vi "Facade.vi"(0 "Data In":T4, 2 "Display State In":T2, 3 "Container State":T3) -> (6 "Data Out":T4, 7 "Display State Out":T2, 8 "Action":T1)   [LabVIEW 2015, in "Tone (G3).xctl"]
uses:
  Tone (G3).xctl
  Tone.Properties.ctl
  <vilib>/_xctls/Container State.ctl
  State.ctl
  Utility VIs/Controls/KNumeric (DBL)/KNumeric (DBL).xctl
  Utility VIs/Controls/KCheckbox/KCheckbox.xctl
  <vilib>/_xctls/Action.ctl
  <vilib>/_xctls/XControlSupport.lvlib
panel:
  in  "Random phase":bool(xcontrol)
  in  "Frequency (kHz)":dbl(xcontrol)
  in  "Phase (cycles)":dbl(xcontrol)
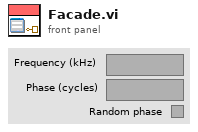
[diagram p1: front panel]
types:
  T1 = typedef "XControlSupport.lvlib/Action.ctl" = cluster{"Data Changed?":bool, "State Changed?":bool, "Action Name":string}
  T2 = typedef "Tone (G3).xctl/State.ctl" = cluster{"enable menu":bool, "ctls":cluster{"Freq":refnum<vi>, "Phase":refnum<vi>, "Random":refnum<vi>}}
  T3 = typedef "XControlSupport.lvlib/Container State.ctl" = cluster{"Indicator?":bool, "Run Mode?":bool, " Refnum":refnum<vi>}
  T4 = typedef "Tone (G3).xctl/Tone.Properties.ctl" = cluster{"Frequency (kHz)":dbl, "Phase (cycles)":dbl, "Random phase":bool}
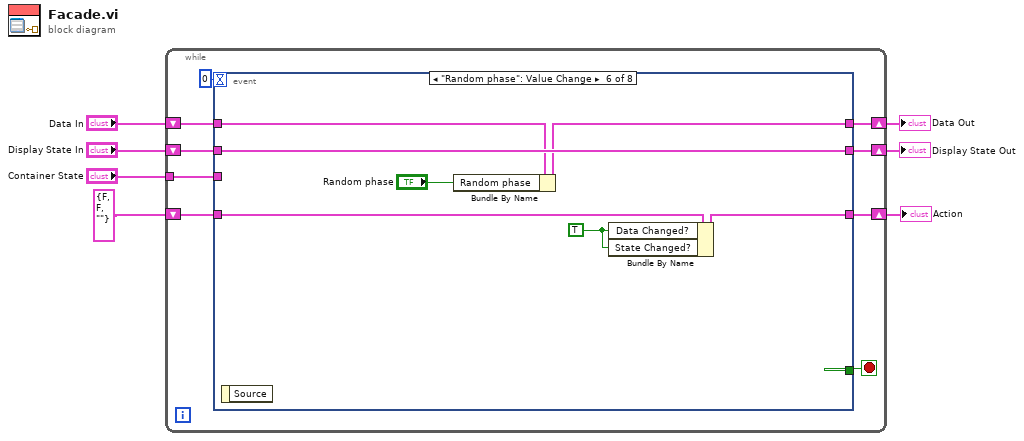
[diagram p0: block diagram]
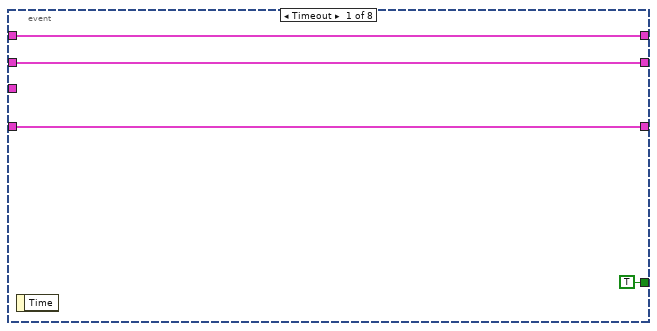
[diagram p2: hidden frame]
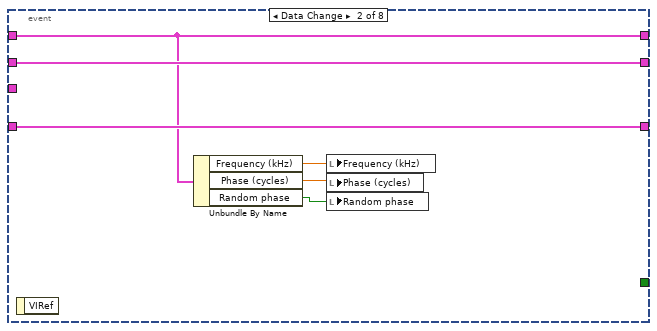
[diagram p3: hidden frame]
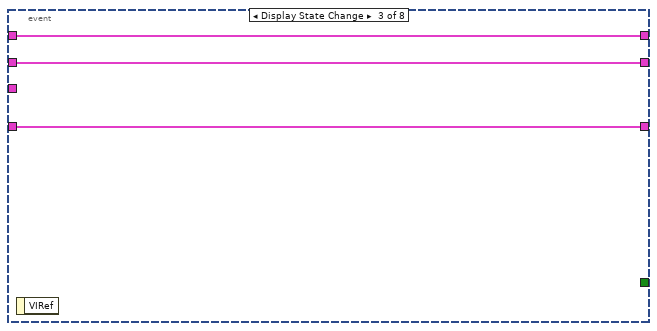
[diagram p4: hidden frame]
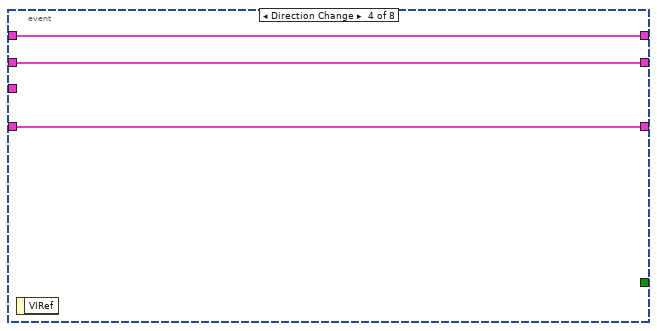
[diagram p5: hidden frame]
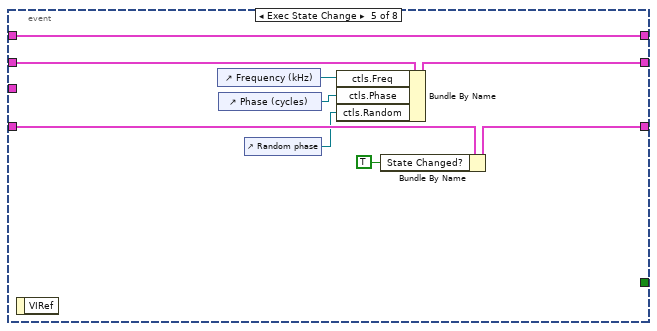
[diagram p6: hidden frame]
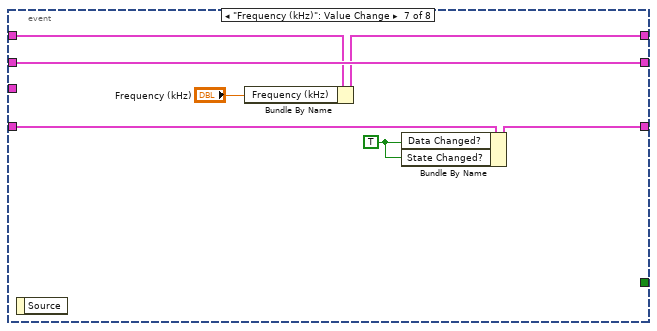
[diagram p7: hidden frame]
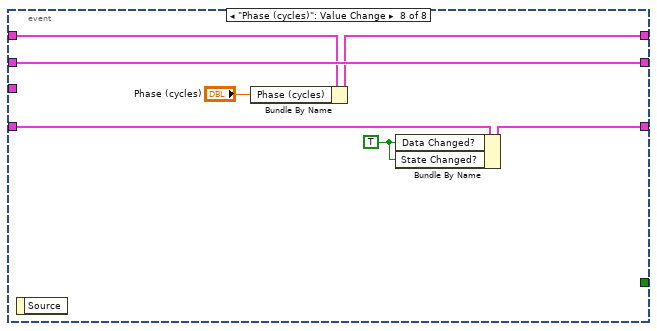
[diagram p8: hidden frame]
diagram:
  n1 = while {
    shift-right: [w15] -> w4
    shift-left: "Display State In" -> [w16]
    tunnel: "Container State" -> [w12]
    shift-right: [w10] -> w7
    shift-left: "Data In" -> [w11]
    shift-right: [w8] -> w2
    shift-left: T1 {"Data Changed?"=FALSE, "State Changed?"=FALSE, "Action Name"=""} ("Action") -> [w9]
    stop <- w14 stop-if-true
    n2 = event shown="[5] \"Random phase\": Value Change" {
      selector: _ -> [_ _ _ _ _ _ _ _]
      dyn-events: _ -> [_ _ _ _ _ _ _ _]
      timeout: 0 -> [_ _ _ _ _ _ _ _]
      tunnel: w16 -> [w18 w26 w27 w32 w41 w48 w55 w62]
      tunnel: [w18 w26 w27 w32 w38 w48 w55 w62] -> w15
      tunnel: [TRUE _ _ _ _ _ _ _] -> w14
      tunnel: w12 -> [_ _ _ _ _ _ _ _]
      tunnel: w11 -> [w17 w24 w29 w31 w40 w47 w54 w61]
      tunnel: [w17 w24 w29 w31 w40 w45 w52 w59] -> w10
      tunnel: [w19 w25 w28 w30 w37 w44 w51 w58] -> w8
      tunnel: w9 -> [w19 w25 w28 w30 w39 w46 w53 w60]
      event Timeout {
        n3 = event-data() -> ()  [unwired: 1 in, 1 out]
      }
      event Data Change {
        n4 = event-data() -> ()  [unwired: 1 in, 1 out]
        n5 = Unbundle By Name(w24) -> ("Frequency (kHz)"=w23:dbl, "Phase (cycles)"=w22:dbl, "Random phase"=w21:bool)
        n6 = local write "Frequency (kHz)"(w23) -> ()
        n7 = local write "Phase (cycles)"(w22) -> ()
        n8 = local write "Random phase"(w21) -> ()
      }
      event Display State Change {
        n9 = event-data() -> ()  [unwired: 1 in, 1 out]
      }
      event Direction Change {
        n10 = event-data() -> ()  [unwired: 1 in, 1 out]
      }
      event Exec State Change {
        n11 = event-data() -> ()  [unwired: 1 in, 1 out]
        n12 = control-ref of="Frequency (kHz)"() -> (w35:refnum<vi>)
        n13 = control-ref of="Phase (cycles)"() -> (w34:refnum<vi>)
        n14 = control-ref of="Random phase"() -> (w33:refnum<vi>)
        n15 = Bundle By Name(cluster=w41, "ctls.Freq"=w35, "ctls.Phase"=w34, "ctls.Random"=w33) -> (w38:T2)
        n16 = Bundle By Name(cluster=w39, "State Changed?"=TRUE) -> (w37:T1)
      }
      event "Random phase": Value Change {
        w42 = TRUE ("Data Changed?")
        n17 = event-data() -> ()  [unwired: 1 in, 1 out]
        n18 = Bundle By Name(cluster=w47, "Random phase"="Random phase") -> (w45:T4)
        n19 = Bundle By Name(cluster=w46, "Data Changed?"=w42, "State Changed?"=w42) -> (w44:T1)
      }
      event "Frequency (kHz)": Value Change {
        w49 = TRUE ("Data Changed?")
        n20 = event-data() -> ()  [unwired: 1 in, 1 out]
        n21 = Bundle By Name(cluster=w54, "Frequency (kHz)"="Frequency (kHz)") -> (w52:T4)
        n22 = Bundle By Name(cluster=w53, "Data Changed?"=w49, "State Changed?"=w49) -> (w51:T1)
      }
      event "Phase (cycles)": Value Change {
        w56 = TRUE ("Data Changed?")
        n23 = event-data() -> ()  [unwired: 1 in, 1 out]
        n24 = Bundle By Name(cluster=w61, "Phase (cycles)"="Phase (cycles)") -> (w59:T4)
        n25 = Bundle By Name(cluster=w60, "Data Changed?"=w56, "State Changed?"=w56) -> (w58:T1)
      }
    }
  }
  "Display State Out" <- w4
  "Data Out" <- w7
  "Action" <- w2
